vi "Cal Inst - Number of Phases.vi"(8 "error in":errorcluster, 11 "Hardware Resources in":T1={"VISA Refnum in"="", "Serial Configuration"={"Baud Rate"=460800, "Flow Control"=0}, "Voltage Level (0V)"=0.0, "Output Phase(s) (1-Phase)"=0, "Active Phase (1:Phase 1)"=1, "Naked Sphere Phase"=1, "Insulated Sphere Phase"=2} {"Insulated Sphere Phase" items=["Phase 1"=1, "Phase 2"=2, "Phase 3"=3]; "Naked Sphere Phase" items=["Phase 1"=1, "Phase 2"=2, "Phase 3"=3]; "Output Phase(s) (1-Phase)" items=["3 phase", "1 phase"]; "Active Phase (1:Phase 1)" items=["Phase 1"=1, "Phase 2"=2, "Phase 3"=3]; "Serial Configuration"."Flow Control" items=["None", "XON/XOFF", "RTS/CTS", "XON/XOFF & RTS/CTS", "DTR/DSR", "XON/XOFF & DTR/DSR"]; "Serial Configuration"."Baud Rate" items=["9600"=9600, "19200"=19200, "38400"=38400, "57600"=57600, "115200"=115200, "230400"=230400, "460800"=460800]}) -> (0 "error out":errorcluster, 3 "Hardware Resources out":T1={"VISA Refnum in"="", "Serial Configuration"={"Baud Rate"=460800, "Flow Control"=0}, "Voltage Level (0V)"=0.0, "Output Phase(s) (1-Phase)"=0, "Active Phase (1:Phase 1)"=1, "Naked Sphere Phase"=1, "Insulated Sphere Phase"=2} {"Insulated Sphere Phase" items=["Phase 1"=1, "Phase 2"=2, "Phase 3"=3]; "Naked Sphere Phase" items=["Phase 1"=1, "Phase 2"=2, "Phase 3"=3]; "Output Phase(s) (1-Phase)" items=["3 phase", "1 phase"]; "Active Phase (1:Phase 1)" items=["Phase 1"=1, "Phase 2"=2, "Phase 3"=3]; "Serial Configuration"."Flow Control" items=["None", "XON/XOFF", "RTS/CTS", "XON/XOFF & RTS/CTS", "DTR/DSR", "XON/XOFF & DTR/DSR"]; "Serial Configuration"."Baud Rate" items=["9600"=9600, "19200"=19200, "38400"=38400, "57600"=57600, "115200"=115200, "230400"=230400, "460800"=460800]})   [LabVIEW 2013, in "Cal Inst.lvlib" / "Cal Inst Acquisition.lvlib"]
uses:
  Acquisition/Cal Inst Acquisition.lvlib
  Acquisition/Hardware Configuration.ctl
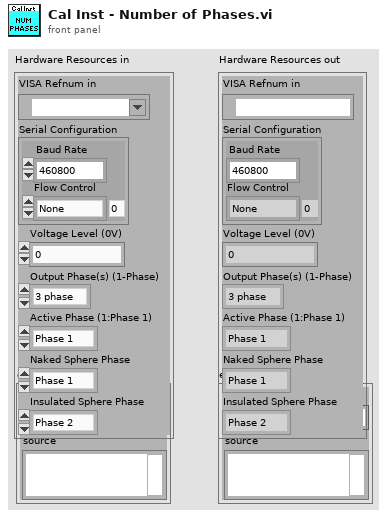
[diagram p1: front panel]
types:
  T1 = typedef "Cal Inst.lvlib/Cal Inst Acquisition.lvlib/Hardware Configuration.ctl" = cluster{"VISA Refnum in":refnum<visa-resource-name>, "Serial Configuration":cluster{"Baud Rate":u32, "Flow Control":u16}, "Voltage Level (0V)":dbl, "Output Phase(s) (1-Phase)":u16, "Active Phase (1:Phase 1)":i32, "Naked Sphere Phase":i32, "Insulated Sphere Phase":i32}
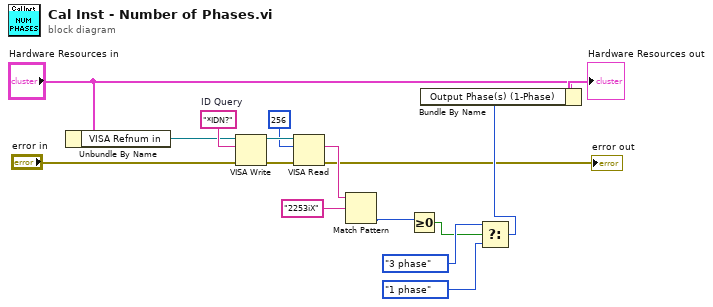
[diagram p0: block diagram]
diagram:
  w12 = "*IDN?"  # ID Query
  n1 = Unbundle By Name("Hardware Resources in") -> ("VISA Refnum in"=w1:refnum<visa-resource-name>)
  n2 = VISA Write(VISA resource name=w1, write buffer=w12, error in (no error)="error in") -> (VISA resource name out=w15:refnum<visa-resource-name>, error out=w14:errorcluster)  [unwired: 1 out]
  n3 = VISA Read(VISA resource name=w15, byte count=u32 256, error in (no error)=w14) -> (read buffer=w9:string, error out=→"error out":errorcluster)  [unwired: 2 out]
  n4 = Match Pattern(string=w9, regular expression="2253iX") -> (offset past match=w11:i32)  [unwired: 1 in, 3 out]
  n5 = Greater Or Equal To 0?(x=w11) -> (x >= 0?=w7:bool)
  n6 = Select(t=enum16{"3 phase", "1 phase"}."3 phase" ("Number of Phases"), s=w7, f=enum16{"3 phase", "1 phase"}."1 phase" ("Number of Phases")) -> (s? t:f=w5:enum16{"3 phase", "1 phase"})
  n7 = Bundle By Name(cluster="Hardware Resources in", "Output Phase(s) (1-Phase)"=w5) -> (→"Hardware Resources out":T1)
